vi "Init Event Handler.vi"(8 "error in (no error)":errorcluster, 11 "VolatusCoreTask in":refnum<class "VolatusCoreTask.lvclass">) -> (0 "error out":errorcluster, 3 "VolatusCoreTask out":refnum<class "VolatusCoreTask.lvclass">)   [LabVIEW 2020, in "Volatus.lvlib" / "VolatusCoreTask.lvclass"]
uses:
  VolatusCoreTask.lvclass
  C:/Program Files (x86)/National Instruments/LabVIEW 2020/vi.lib/ActorFramework/Actor/Actor.lvclass
  C:/dev/lv20CE/relink/lv-volatus/Volatus/Task/Task.lvclass
  VolatusCoreTask.lvclass/VolatusCoreTask.ctl
  Event API/EventAPI.lvclass/EventAPI.ctl
  EventHandler Messages/Handle Event Msg/Handle Event Msg.lvclass/Handle Event Msg.ctl
  <vilib>/ActorFramework/Message Enqueuer/Message Enqueuer.lvclass/Message Enqueuer.ctl
  EventHandler Messages/Handle Event Msg/Send Handle Event.vi
  <vilib>/ActorFramework/Message Enqueuer/Enqueue.vi
  EventHandlerTask/EventHandlerTask.lvclass
  EventHandler Messages/Handle Event Msg/Handle Event Msg.lvclass
  C:/Program Files (x86)/National Instruments/LabVIEW 2020/vi.lib/ActorFramework/Message/Message.lvclass
  <vilib>/ActorFramework/Message Priority Queue/Priority Enqueue.vi
  Task/Set Core APIs.vi
  App/App.lvclass
  Event API/EventAPI.lvclass
  <vilib>/ActorFramework/Actor/Actor.lvclass
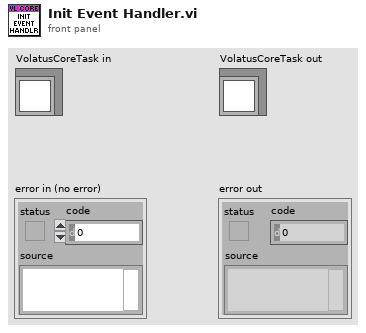
[diagram p1: front panel]
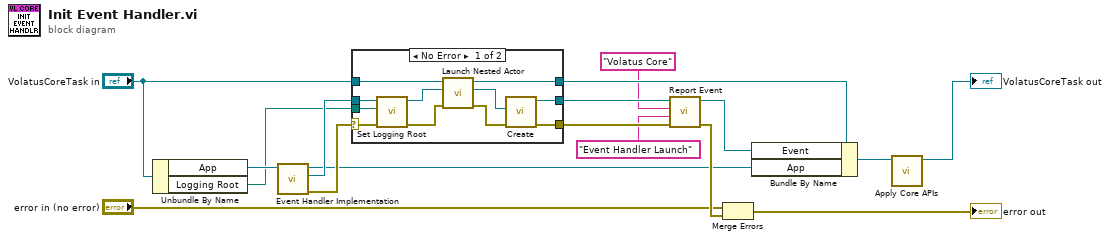
[diagram p0: block diagram]
diagram:
  n1 = Unbundle By Name("VolatusCoreTask in") -> ("App"=w15:refnum<class "App.lvclass">, "Logging Root"=w13:path)
  n2 = call-dynamic "Event Handler Implementation.vi"("App in"=w15) -> ("error out"=w16:errorcluster, "EventHandlerTask"=w14:refnum<class "EventHandlerTask.lvclass">, "App out"=w12:refnum<class "App.lvclass">)  [unwired: 8 in]
  n3 = case shown="No Error" w16 {
    selector: w16 -> [w24 w30]
    tunnel: w14 -> [w28 _]
    tunnel: w13 -> [w27 _]
    tunnel: "VolatusCoreTask in" -> [w26 w29]
    tunnel: [w20 w29] -> w9
    tunnel: [w19 _] -> w8
    tunnel: [w18 w30] -> w3
    frame No Error {
      n4 = call-dynamic "Set Logging Root.vi"("error in (no error)"=w24, "Logging Root"=w27, "EventHandler in"=w28) -> ("error out"=w23:errorcluster, "EventHandler out"=w25:refnum<class "EventHandlerTask.lvclass">)  [unwired: 7 in]
      n5 = call <vilib>:"Launch Nested Actor.vi"("error in (no error)"=w23, "Nested Actor"=w25, "Caller Actor in"=w26) -> ("error out"=w21:errorcluster, "Nested Actor's Enqueuer"=w22:refnum<class "Message Enqueuer.lvclass">, "Caller Actor out"=w20:refnum<class "VolatusCoreTask.lvclass">)  [unwired: 6 in]
      n6 = call "Create.vi"("error in (no error)"=w21, "EnQr"=w22) -> ("error out"=w18:errorcluster, "Event API out"=w19:refnum<class "EventAPI.lvclass">)  [unwired: 8 in]
    }
    frame Error {
    }
  }
  n7 = call "Report Event.vi"("error in (no error)"=w3, "Message"="Event Handler Launch", "Context"="Volatus Core", "Event API in"=w8) -> ("error out"=w17:errorcluster, "Event API out"=w5:refnum<class "EventAPI.lvclass">)  [unwired: 6 in]
  n8 = Merge Errors("error in (no error)", w17) -> (→"error out":errorcluster)
  n9 = Bundle By Name(cluster=w9, "Event"=w5, "App"=w12) -> (w11:refnum<class "VolatusCoreTask.lvclass">)
  n10 = call "Apply Core APIs.vi"("VolatusCoreTask in"=w11) -> ("VolatusCoreTask out"=→"VolatusCoreTask out":refnum<class "VolatusCoreTask.lvclass">)  [unwired: 9 in, 1 out]
